vi "Self-Sort.vi"(7 "SubComponent List":refnum<class "1553 SubComponent.lvclass">[](array[class]), 8 "error in (no error)":errorcluster, 11 "Bus Monitor in":refnum<class "Bus Monitor.lvclass">) -> (0 "error out":errorcluster, 5 "SubComponent List out":refnum<class "1553 SubComponent.lvclass">[](array[class]))   [LabVIEW 2016, in "BCI-1553 API.lvlib" / "Bus Monitor.lvclass"]
doc: "<DO NOT CALL>\n\nVirtual: All the children who decide to implement this will need to provide a means for locating themselves in the SubComonent List and updating their location appropriately."
uses:
  Bus Monitor.lvclass
  1553 SubComponent/1553 SubComponent.lvclass
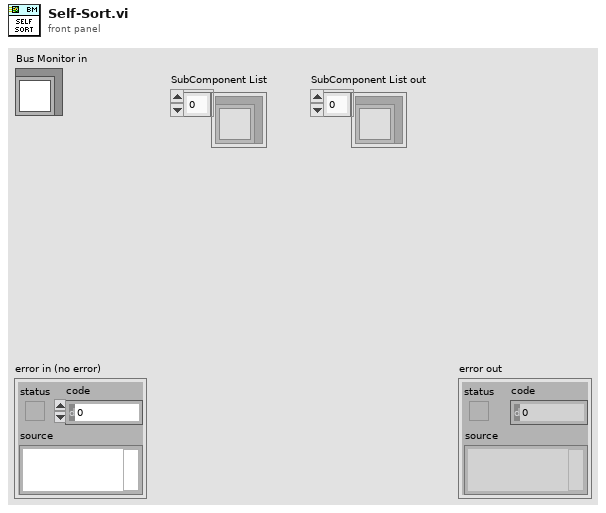
[diagram p1: front panel]
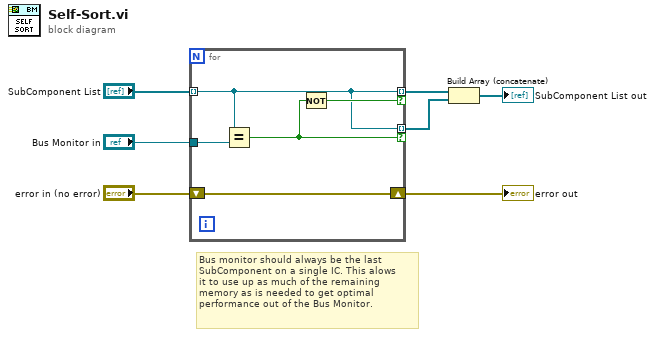
[diagram p0: block diagram]
diagram:
  # "Bus monitor should always be the last\nSubComponent on a single IC. This alows\nit to use up as much of the remaining \nmemory as is needed to get optimal\nperformance out of the Bus Monitor."
  n1 = for {
    shift-right: [w12] -> w7
    shift-left: "error in (no error)" -> [w12]
    tunnel: "Bus Monitor in" -> [w11]
    tunnel: "SubComponent List" -> [w9] mode=indexing
    tunnel: [w9] -> w2 mode=indexing if=w10
    tunnel: [w9] -> w3 mode=indexing if=w8
    n2 = Equal?(x=w9, y=w11) -> (x = y?=w8:bool)
    n3 = Not(x=w8) -> (.not. x?=w10:bool)
  }
  "error out" <- w7
  n4 = Build Array (concatenate)(w2, w3) -> (→"SubComponent List out":refnum<class "1553 SubComponent.lvclass">[])
